vi "SW_Create_density_overlay.vi"(2 "Background color":u32, 3 "Density histogram":u32[][](array[numeric]), 4 "Diagram with zones":u32[][](array[numeric]), 5 "Diagram no zones":u32[][](array[numeric])) -> (0 "Density map with zones":u32[][](array[numeric]), 1 "Density map no zones":u32[][](array[numeric]))   [LabVIEW 2016]
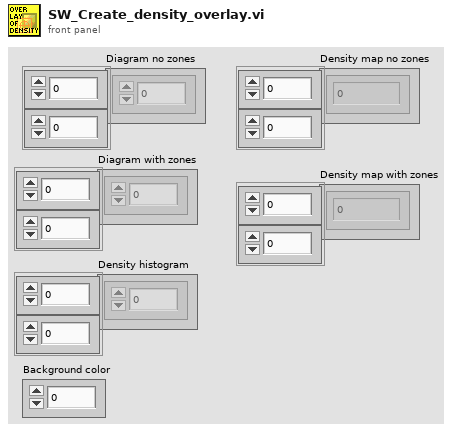
[diagram p1: front panel]
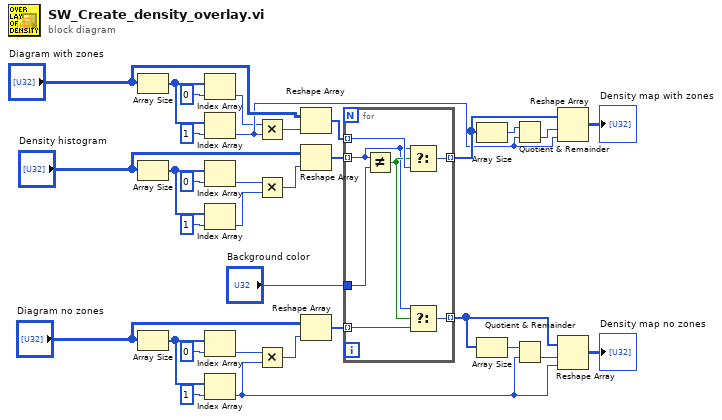
[diagram p0: block diagram]
diagram:
  n1 = Array Size(array="Diagram with zones") -> (size(s)=w18:i32[])
  n2 = Array Size(array="Density histogram") -> (size(s)=w13:i32[])
  n3 = Array Size(array="Diagram no zones") -> (size(s)=w7:i32[])
  n4 = Index Array(array=w18, index=0) -> (element=w19:i32)
  n5 = Index Array(array=w18, index=1) -> (element=w21:i32)
  n6 = Index Array(array=w13, index=0) -> (element=w12:i32)
  n7 = Index Array(array=w13, index=1) -> (element=w11:i32)
  n8 = Index Array(array=w7, index=0) -> (element=w8:i32)
  n9 = Index Array(array=w7, index=1) -> (element=w22:i32)
  n10 = Multiply(x=w19, y=w21) -> (x*y=w20:i32)
  n11 = Multiply(x=w12, y=w11) -> (x*y=w10:i32)
  n12 = Multiply(x=w8, y=w22) -> (x*y=w9:i32)
  n13 = Reshape Array("Diagram with zones", w20) -> (w25:u32[])
  n14 = Reshape Array("Density histogram", w10) -> (w27:u32[])
  n15 = Reshape Array("Diagram no zones", w9) -> (w28:u32[])
  n16 = for {
    tunnel: w27 -> [w34] mode=indexing
    tunnel: w25 -> [w40] mode=indexing
    tunnel: [w39] -> w23 mode=indexing
    tunnel: "Background color" -> [w38]
    tunnel: w28 -> [w37] mode=indexing
    tunnel: [w36] -> w24 mode=indexing
    n17 = Not Equal?(x=w34, y=w38) -> (x != y?=w35:bool)
    n18 = Select(t=w34, s=w35, f=w40) -> (s? t:f=w39:u32)
    n19 = Select(t=w34, s=w35, f=w37) -> (s? t:f=w36:u32)
  }
  n20 = Array Size(array=w23) -> (size(s)=w3:i32)
  n21 = Array Size(array=w24) -> (size(s)=w2:i32)
  n22 = Quotient & Remainder(x=w3, y=w21) -> (floor(x/y)=w4:i32)  [unwired: 1 out]
  n23 = Quotient & Remainder(x=w2, y=w22) -> (floor(x/y)=w1:i32)  [unwired: 1 out]
  n24 = Reshape Array(w23, w4, w21) -> (→"Density map with zones":u32[][])
  n25 = Reshape Array(w24, w1, w22) -> (→"Density map no zones":u32[][])
